vi "Update Status Table.vi"(8 "error in (no error)":errorcluster, 10 "Plugin Filter":string, 11 "CIFManager_UI in":refnum<class "CIF_UI.lvclass">) -> (0 "error out":errorcluster)   [LabVIEW 2021, in "CIF_UI.lvclass"]
uses:
  CIF_UI.lvclass
  CIF_UI.lvclass/CIF_UI.ctl
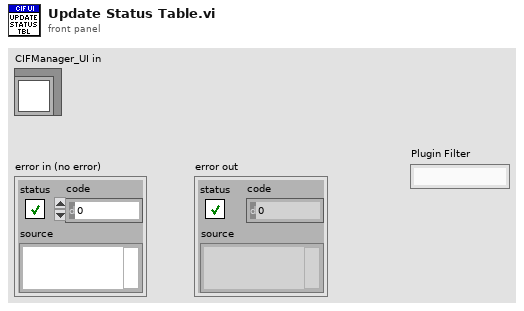
[diagram p1: front panel]
types:
  T1 = typedef "CIF_UI.lvclass/Plugin Connection Map.ctl" = map{string, T2}
  T2 = typedef "CIF_UI.lvclass/Plugin Connections.ctl" = cluster{"gRPC ID":T3, "Plugin Info":T4}
  T3 = typedef "grpc-lvsupport-release.lvlib/grpcId.ctl" = u64
  T4 = typedef "CIF_UI.lvclass/PluginInfo.ctl" = cluster{"Name":string, "Type":string, "grpc_port":i32, "Version":T5, "Node Status":T6}
  T5 = typedef "CIF_UI.lvclass/Version.ctl" = cluster{"Major":i32, "Minor":i32, "Fix":i32}
  T6 = typedef "CIFCoreCommon.lvlib/gRPC Reported Plugin Status.ctl" = cluster{"State":T7, "Timing Statistics (us)":T8, "FIFO Statistics (us)":T10, "error":T11, "Monitor Doubles":T12, "Monitor U64":T13, "Monitor I64":T14}
  T7 = typedef "CIFCoreCommon.lvlib/Plugin State.ctl" = enum32{"Null", "Creating", "Listening", "Running", "CleaningUp", "Destroying"}
  T8 = typedef "CIFCoreCommon.lvlib/Timing Statistics.ctl" = cluster{"Period":T9, "Wake Error":T9, "Execute":T9, "Housekeep":T9, "Idle":T9, "Cleanup":T9, "Custom 1 (custom units)":T9, "Custom 2 (custom units)":T9}
  T9 = typedef "CIFCoreCommon.lvlib/Timing Stats Base.ctl" = cluster{"Max":i64, "Avg":dbl, "Min":i64}
  T10 = typedef "CIFCoreCommon.lvlib/FIFO Statistics.ctl" = cluster{"From T0":T9, "From Previous Plugin":T9, "Output Error":T9}
  T11 = typedef "CIFCoreCommon.lvlib/Simple Error.ctl" = cluster{"status":bool, "code":i32}
  T12 = typedef "CIFCoreCommon.lvlib/Monitor Doubles.ctl" = cluster{"1":dbl, "2":dbl, "3":dbl, "4":dbl}
  T13 = typedef "CIFCoreCommon.lvlib/Monitor U64.ctl" = cluster{"1":u64, "2":u64, "3":u64, "4":u64}
  T14 = typedef "CIFCoreCommon.lvlib/Monitor I64.ctl" = cluster{"1":i64, "2":i64, "3":i64, "4":i64}
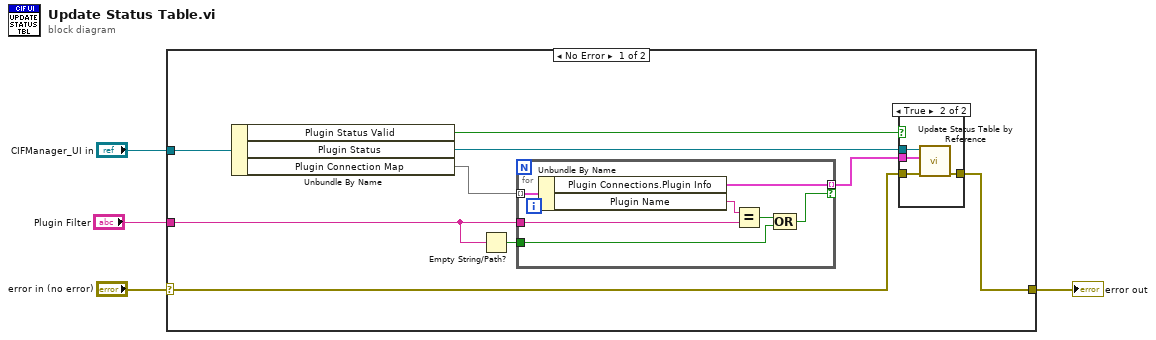
[diagram p0: block diagram]
diagram:
  n1 = case shown="No Error" "error in (no error)" {
    selector: "error in (no error)" -> [w10 w26]
    tunnel: [w13 w26] -> w3
    tunnel: "CIFManager_UI in" -> [w9 _]
    tunnel: "Plugin Filter" -> [w6 _]
    frame No Error {
      n2 = Unbundle By Name(w9) -> ("Plugin Status Valid"=w8:bool, "Plugin Status"=w12:refnum<vi>, "Plugin Connection Map"=w11:T1)
      n3 = Empty String/Path?(string/path=w6) -> (empty?=w5:bool)
      n4 = for {
        tunnel: w11 -> [w20] mode=indexing
        tunnel: [w19] -> w7 mode=indexing if=w14
        tunnel: w6 -> [w18]
        tunnel: w5 -> [w15]
        n5 = Unbundle By Name(w20) -> ("Plugin Connections.Plugin Info"=w19:T4, "Plugin Name"=w17:string)
        n6 = Equal?(x=w17, y=w18) -> (x = y?=w16:bool)
        n7 = Compound Arithmetic op=OR(w16, w15) -> (w14:bool)
      }
      n8 = case shown="True" w8 {
        tunnel: [w21 w25] -> w13
        tunnel: w12 -> [_ w24]
        tunnel: w7 -> [_ w23]
        tunnel: w10 -> [w21 w22]
        frame False {
        }
        frame True {
          n9 = call "Update Status Table by Reference.vi"("error in (no error)"=w22, "Plugin Info Array"=w23, "Table Control in"=w24) -> ("error out"=w25:errorcluster)  [unwired: 8 in]
        }
      }
    }
    frame Error {
    }
  }
  "error out" <- w3
